vi "ClusterWayToSendServerSide.vi"() -> ()   [LabVIEW 2019]
panel:
  out "error out":errorcluster
  out "bytes written":i32
  in  "stop from Server Side":bool
  in  "Full Name":string
  in  "Is Single":bool
  in  "Age":dbl
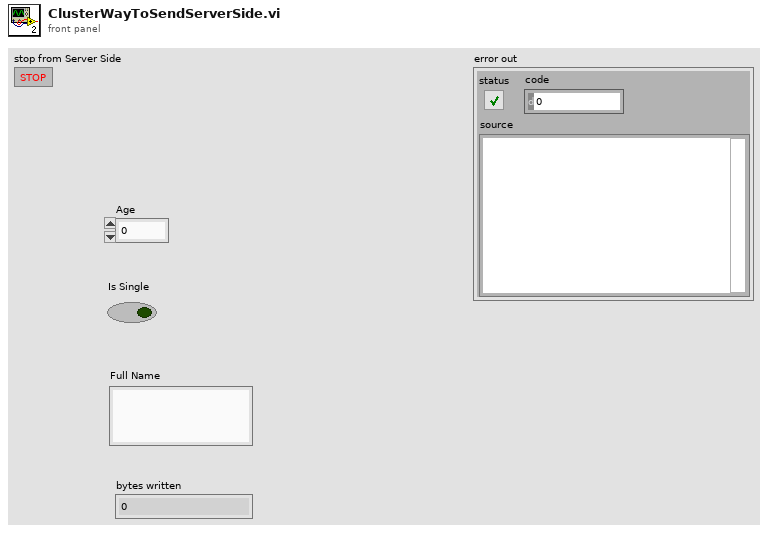
[diagram p1: front panel]
types:
  T1 = cluster{"Age ":dbl, "Is Single ":bool, "Full Name ":string}
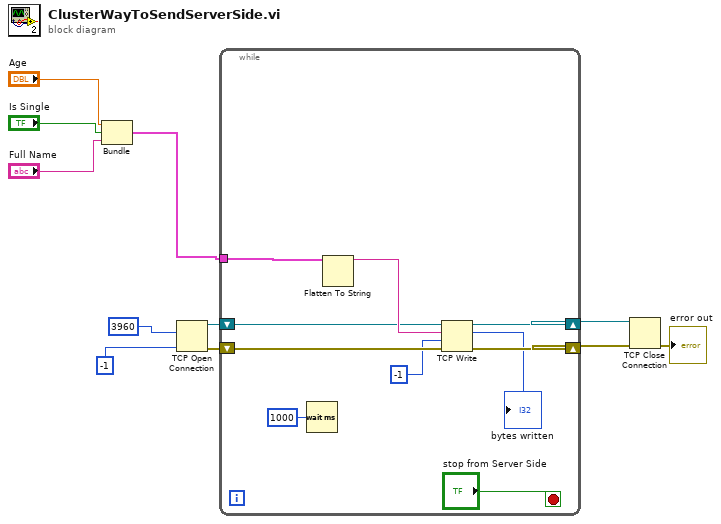
[diagram p0: block diagram]
diagram:
  n1 = Bundle("Age"="Age", "Is Single"="Is Single", "Full Name"="Full Name") -> (w2:T1)  [unwired: 1 in]
  n2 = TCP Open Connection(remote port or service name=u16 3960, timeout ms (60000)=-1) -> (connection ID=w5:refnum<k5>, error out=w6:errorcluster)  [unwired: 3 in]
  n3 = while {
    shift-right: [w18] -> w11
    shift-left: w5 -> [w20]
    shift-right: [w17] -> w10
    shift-left: w6 -> [w19]
    tunnel: w2 -> [w16]
    stop <- "stop from Server Side" stop-if-true
    n4 = Wait (ms)(milliseconds to wait=u32 1000) -> ()  [unwired: 1 out]
    n5 = Flatten To String(anything=w16) -> (data string=w21:string)  [unwired: 3 in, 2 out]
    n6 = TCP Write(connection ID=w20, data in=w21, error in (no error)=w19, 9:-1 ("timeout ms (25000)")) -> (connection ID out=w18:refnum<k5>, bytes written=→"bytes written":i32, error out=w17:errorcluster)
  }
  n7 = TCP Close Connection(connection ID=w11, error in (no error)=w10) -> (error out=→"error out":errorcluster)  [unwired: 1 in, 1 out]
